vi "acq.ImageAccumulator.EL.vi"(6 "loop":i32, 8 "error in":errorcluster, 10 "EL in":u16[][](array[numeric])) -> (0 "error out":errorcluster, 2 "EL out":u16[][](array[numeric]))   [LabVIEW 2020]
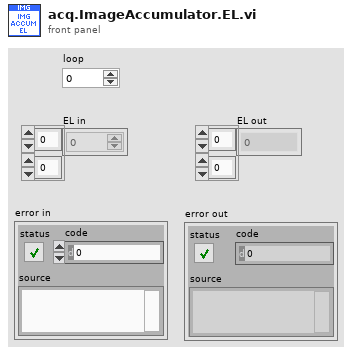
[diagram p1: front panel]
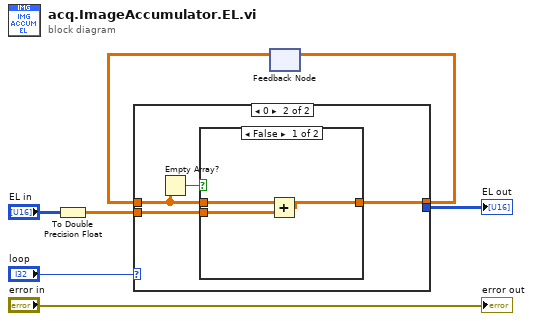
[diagram p0: block diagram]
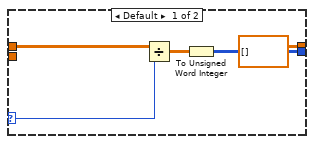
[diagram p2: hidden frame]
diagram:
  n1 = To Double Precision Float(number="EL in") -> (double precision float=w5:dbl[][])
  n2 = feedback #1() -> (w3:dbl[][])  [unwired: 1 in]
  n3 = case shown="0" "loop" {
    selector: "loop" -> [w8 _]
    tunnel: w3 -> [w12 w13]
    tunnel: w5 -> [_ w14]
    tunnel: [dbl[][] [] w16] -> w4
    tunnel: [w10 _] -> w2
    frame Default {
      n4 = Divide(x=w12, y=w8) -> (x/y=w11:dbl[][])
      n5 = To Unsigned Word Integer(number=w11) -> (unsigned 16bit integer=w10:u16[][])
    }
    frame 0 {
      n6 = Empty Array?(array=w13) -> (empty?=w15:bool)
      n7 = case shown="False" w15 {
        tunnel: w13 -> [w19 _]
        tunnel: w14 -> [w18 w20]
        tunnel: [w17 w20] -> w16
        frame False {
          n8 = Add(x=w19, y=w18) -> (x+y=w17:dbl[][])
        }
        frame True {
        }
      }
    }
  }
  "EL out" <- w2
  n9 = feedback-in #1(w4) -> ()
  "error out" <- "error in"
